vi "Untitssss.vi"() -> ()   [LabVIEW 2020]
uses:
  <vilib>/Instr/_visa.llb/VISA Configure Serial Port (Instr).vi
panel:
  in  "write buffer":string
  in  "开关":bool=TRUE
  out "错误输出":cluster{"status":bool, i32, string}={"status"=FALSE, 1073676294, "VISA Read in Untitled 1.vi"}
  in  "串口":refnum<visa-resource-name>="COM4"
  in  "串口设置":T1={"流控制 (0:none)"=0, "停止位 (10: 1 bit)"=10, "奇偶校验 (0:none)"=0, "数据比特 (8)"=8, "比特率 (115200)"=115200} {"数据比特 (8)" min=5 max=8 step=1; "奇偶校验 (0:none)" items=["None", "Odd", "Even", "Mark", "Space"]; "流控制 (0:none)" items=["None", "XON/XOFF", "RTS/CTS", "XON/XOFF & RTS/CTS", "DTR/DSR", "XON/XOFF & DTR/DSR"]}
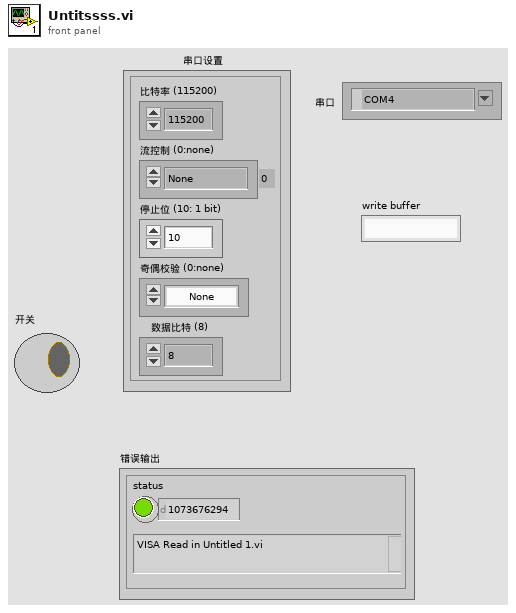
[diagram p1: front panel]
types:
  T1 = cluster{"流控制 (0:none)":u16, "停止位 (10: 1 bit)":u16, "奇偶校验 (0:none)":u16, "数据比特 (8)":u16, "比特率 (115200)":u32}
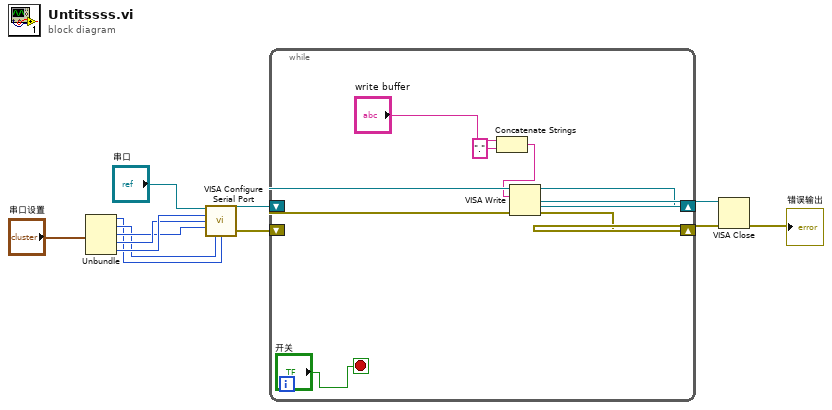
[diagram p0: block diagram]
diagram:
  n1 = Unbundle("串口设置") -> ("流控制 (0:none)"=w4:u16, "停止位 (10: 1 bit)"=w5:u16, "奇偶校验 (0:none)"=w6:u16, "数据比特 (8)"=w7:u16, "比特率 (115200)"=w8:u32)
  n2 = call-poly "VISA Configure Serial Port"("VISA resource name"="串口", "baud rate (9600)"=w8, "data bits (8)"=w7, "parity (0:none)"=w6, "stop bits (10: 1 bit)"=w5, "flow control (0:none)"=w4) -> ("VISA resource name out"=w12:refnum<visa-resource-name>, "error out"=w11:errorcluster)  [unwired: 8 in]
  n3 = while {
    shift-right: [w17] -> w2
    shift-left: w12 -> [w19]
    shift-right: [w16] -> w3
    shift-left: w11 -> [w18]
    stop <- "开关" stop-if-true
    n4 = Concatenate Strings("write buffer", "." ("string")) -> (w13:string)
    n5 = VISA Write(VISA resource name=w19, write buffer=w13, error in (no error)=w18) -> (VISA resource name out=w17:refnum<visa-resource-name>, error out=w16:errorcluster)  [unwired: 1 out]
  }
  n6 = VISA Close(VISA resource name=w2, error in (no error)=w3) -> (error out=→"错误输出":errorcluster)
